vi "Comprimir_a_1_archivo.vi"(1 "Acel_paths":path[](array[path])) -> (0 "path_Pasada":path)   [LabVIEW 2015]
panel:
  out "error out":errorcluster
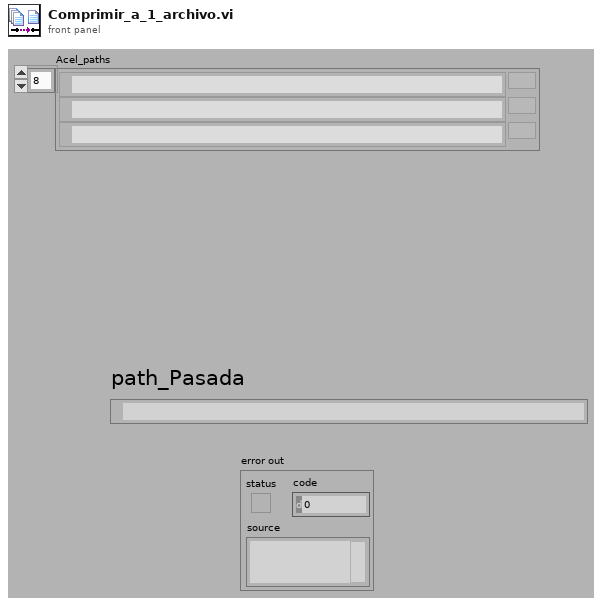
[diagram p1: front panel]
types:
  T1 = enum16{"big-endian, network order", "native, host order", "little-endian"}
  T2 = enum16{"open", "replace", "create", "open or create", "replace or create", "replace or create with confirmation"}
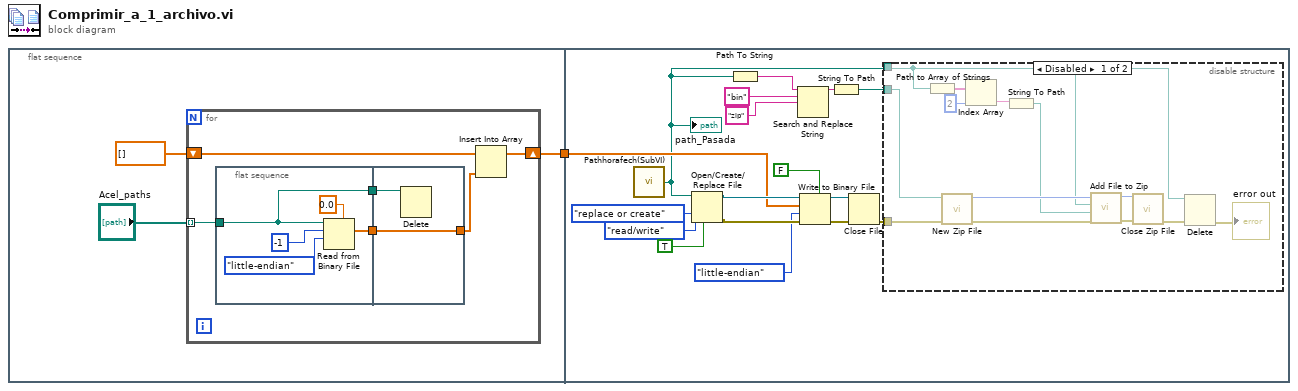
[diagram p0: block diagram]
diagram:
  n1 = flat-sequence {
    tunnel: [w3] -> w1
    tunnel: w1 -> [w27]
    frame #0 {
      n2 = for {
        tunnel: "Acel_paths" -> [w10] mode=indexing
        shift-right: [w8] -> w3
        shift-left: sgl[] [] -> [w9]
        n3 = flat-sequence {
          tunnel: w10 -> [w11]
          tunnel: [w12] -> w6
          tunnel: [w11] -> w5
          tunnel: [w17] -> w7
          tunnel: w6 -> [w17]
          tunnel: w5 -> [w16]
          frame #0 {
            n4 = Read from Binary File(5:sgl 0.0, 9:T1."little-endian" ("byte order (0:big-endian, network order)"), 10:-1 ("count (1)"), 11:w11) -> (2:w12:sgl[])  [unwired: 1 in, 4 out]
          }
          frame #1 {
            n5 = Delete(path (use dialog)=w16) -> ()  [unwired: 4 in, 3 out]
          }
        }
        n6 = Insert Into Array(array=w9, new element=w7) -> (w8:sgl[])  [unwired: 1 in]
      }
    }
    frame #1 {
      n7 = call "Pathhorafech(SubVI).vi"() -> ("path"=w18:path)
      "path_Pasada" <- w18
      n8 = Open/Create/Replace File(file path (use dialog)=w18, operation (0:open)=T2."replace or create", access (0:read/write)=enum16{"read/write", "read-only", "write-only"}."read/write", disable buffering (F)=TRUE) -> (refnum out=w30:refnum<file>, error out=w29:errorcluster)  [unwired: 1 in, 2 out]
      n9 = Path To String(path=w18) -> (string=w23:string)
      n10 = Search and Replace String(input string=w23, search string="bin", replace string="zip" ("replace string (\"\")")) -> (result string=w20:string)  [unwired: 5 in, 3 out]
      n11 = Write to Binary File(file (use dialog)=w30, data=w27, error in=w29, 5:FALSE ("prepend array or string size? (T)"), 9:T1."little-endian" ("byte order (0:big-endian, network order)")) -> (refnum out=w26:refnum<file>, error out=w25:errorcluster)  [unwired: 2 out]
      n12 = String To Path(string=w20) -> (path=w19:path)
      n13 = Close File(refnum=w26, error in=w25) -> (error out=w24:errorcluster)  [unwired: 1 out]
      n14 = disable-structure shown="Disabled" {
        disable-tunnel: w24 -> [w45 _]
        disable-tunnel: w19 -> [w42 _]
        disable-tunnel: w18 -> [w35 _]
        frame Disabled {
          n15 = Path to Array of Strings(0:w35) -> (2:w41:string[])  [unwired: 1 out]
          n16 = call <vilib>:"New Zip File.vi"("error in (no error)"=w45, "target"=w42) -> ("error out"=w44:errorcluster, "zip file out"=w47:i64)  [unwired: 3 in, 1 out]
          n17 = Index Array(array=w41, index=2) -> (element=w39:string)
          n18 = String To Path(string=w39) -> (path=w38:path)
          n19 = call <vilib>:"Add File to Zip.vi"("error in (no error)"=w44, "destination path in zip"=w38, "source file path"=w35, "zip file in"=w47) -> ("error out"=w43:errorcluster, "zip file out"=w46:i64)  [unwired: 6 in]
          n20 = call <vilib>:"Close Zip File.vi"("error in (no error)"=w43, "zip file in"=w46) -> ("error out"=w37:errorcluster)  [unwired: 5 in]
          n21 = Delete(path (use dialog)=w35, error in=w37) -> (error out=→"error out":errorcluster)  [unwired: 3 in, 2 out]
        }
        frame Enabled {
        }
      }
    }
  }
